vi "Teleop Cmd Recieve.vi"(8 "error in (no error)":errorcluster, 10 "Metrics Input":T1, 11 "rt fifo":refnum<k33>) -> (0 "error out":errorcluster, 2 "Updated Drive Metrics":T1)   [LabVIEW 2014]
uses:
  TeleopCmd.ctl
  CmdFlag.ctl
  Drive Train Metrics.ctl
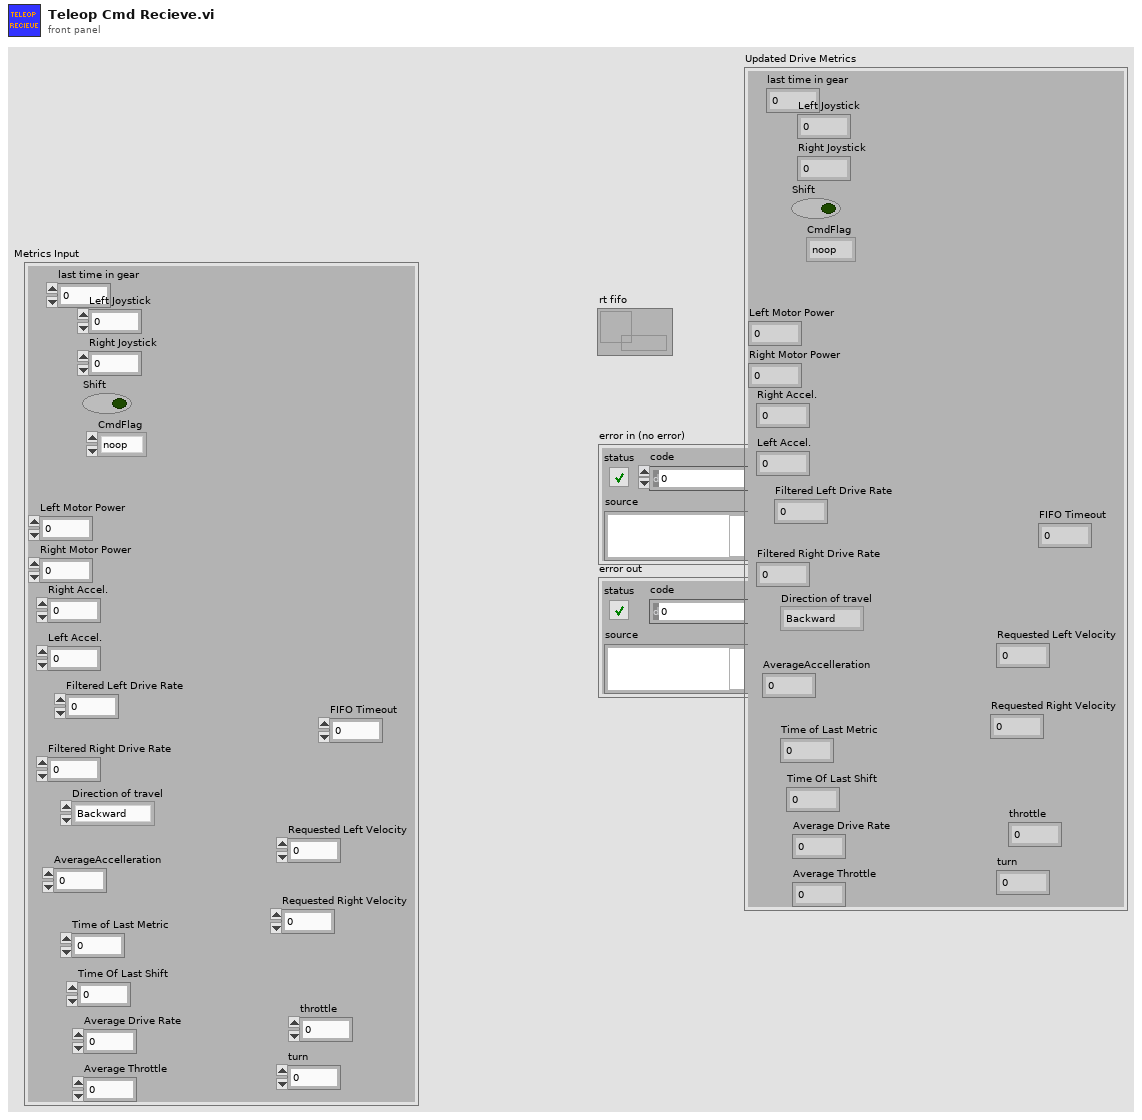
[diagram p1: front panel]
types:
  T1 = typedef "Drive Train Metrics.ctl" = cluster{"last time in gear":u32, "Shift":bool, "Right Joystick":dbl, "Left Joystick":dbl, "CmdFlag":T2, "Right Motor Power":dbl, "Left Motor Power":dbl, "Right Accel.":dbl, "Left Accel.":dbl, "Filtered Left Drive Rate":dbl, "Filtered Right Drive Rate":dbl, "Direction of travel":enum16{"Backward", "Forward", "Spin"}, "AverageAccelleration":dbl, "Time of Last Metric":u32, "Time Of Last Shift":dbl, "Average Drive Rate":dbl, "Average Throttle":dbl, "FIFO Timeout":i32, "Requested Left Velocity":dbl, "Requested Right Velocity":dbl, "throttle":dbl, "turn":dbl}
  T2 = typedef "CmdFlag.ctl" = enum16{"noop", "suspend", "resume"}
  T3 = typedef "TeleopCmd.ctl" = cluster{"Left Joystick":dbl, "Right Joystick":dbl, "Shift":bool, "CmdFlag":T2, "throttle":dbl, "turn":dbl}
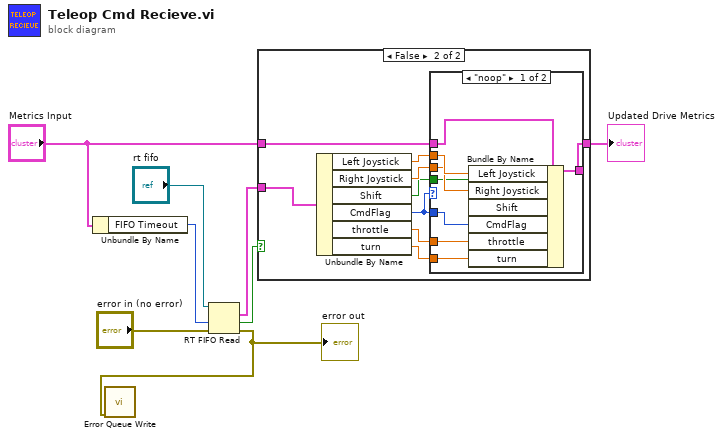
[diagram p0: block diagram]
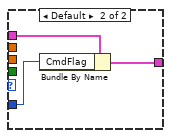
[diagram p3: hidden frame]
diagram:
  n1 = Unbundle By Name("Metrics Input") -> ("FIFO Timeout"=w2:i32)
  n2 = RT FIFO Read(0:"rt fifo", 2:w2, 3:"error in (no error)") -> (9:w6:T3, 10:w4:bool, 11:w1:errorcluster)  [unwired: 1 in, 2 out]
  "error out" <- w1
  n3 = call "Error Queue Write.vi"("error in (no error)"=w1) -> ()  [unwired: 11 in]
  n4 = case shown="False" w4 {
    tunnel: w6 -> [_ w18]
    tunnel: "Metrics Input" -> [w9 w13]
    tunnel: [w9 w12] -> w5
    frame True {
    }
    frame False {
      n5 = Unbundle By Name(w18) -> ("Left Joystick"=w17:dbl, "Right Joystick"=w16:dbl, "Shift"=w15:bool, "CmdFlag"=w14:T2, "throttle"=w11:dbl, "turn"=w10:dbl)
      n6 = case shown="\"noop\"" w14 {
        tunnel: w17 -> [w26 _]
        tunnel: w16 -> [w25 _]
        tunnel: w15 -> [w24 _]
        tunnel: w14 -> [w23 w29]
        tunnel: w13 -> [w22 w28]
        tunnel: [w21 w27] -> w12
        tunnel: w11 -> [w20 _]
        tunnel: w10 -> [w19 _]
        frame "noop" {
          n7 = Bundle By Name(cluster=w22, "Left Joystick"=w26, "Right Joystick"=w25, "Shift"=w24, "CmdFlag"=w23, "throttle"=w20, "turn"=w19) -> (w21:T1)
        }
        frame Default {
          n8 = Bundle By Name(cluster=w28, "CmdFlag"=w29) -> (w27:T1)
        }
      }
    }
  }
  "Updated Drive Metrics" <- w5
